vi "TriggererNot.vi"(10 "Control Name":string="Acquire Trigger", 11 "name or relative path":string="SW-Microscoper.vi") -> (0 "error out":errorcluster, 3 "VI out":refnum<vi>)   [LabVIEW 2012]
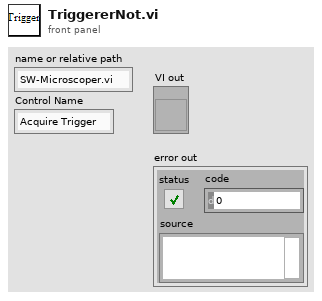
[diagram p1: front panel]
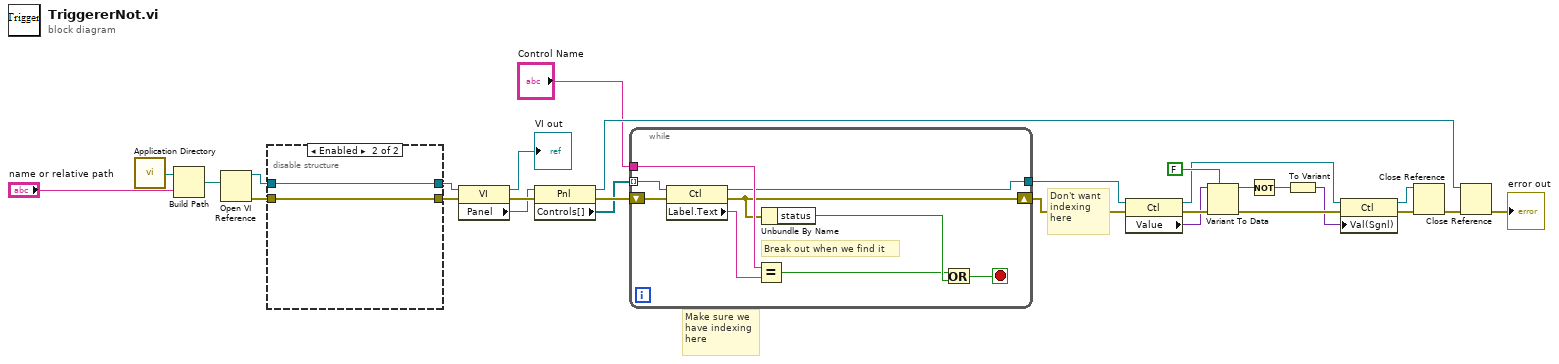
[diagram p0: block diagram]
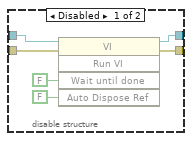
[diagram p2: hidden frame]
diagram:
  # "Don't want\nindexing\nhere"
  # "Make sure we\nhave indexing\nhere"
  n1 = call <vilib>:"Application Directory.vi"() -> ("Application Directory"=w7:path)
  n2 = Build Path(base path=w7, name or relative path="name or relative path") -> (appended path=w6:path)
  n3 = Open VI Reference(vi path=w6) -> (vi reference=w5:refnum<vi>, error out=w4:errorcluster)  [unwired: 5 in]
  n4 = disable-structure shown="Enabled" {
    disable-tunnel: w5 -> [w32 w36]
    disable-tunnel: w4 -> [w31 w35]
    disable-tunnel: [w30 w36] -> w3
    disable-tunnel: [w29 w35] -> w2
    frame Disabled {
      n5 = invoke class="VI" method="Run VI"(reference=w32, error in=w31, "Wait until done"=FALSE ("Front Panel Window:Open"), "Auto Dispose Ref"=FALSE ("Auto Dispose Reference")) -> (reference out=w30:refnum<vi>, error out=w29:errorcluster)  [unwired: 1 in, 3 out]
    }
    frame Enabled {
    }
  }
  n6 = property class="VI"(reference=w3, error in=w2) -> (reference out=→"VI out":refnum<vi>, error out=w21:errorcluster, "Panel"=w9:refnum<vi>)
  n7 = property class="Pnl"(reference=w9, error in=w21) -> (reference out=w28:refnum<vi>, error out=w22:errorcluster, "Controls[]"=w10:refnum<vi>[])
  n8 = while {
    tunnel: w10 -> [w45] mode=indexing
    tunnel: "Control Name" -> [w44]
    tunnel: [w42] -> w11
    shift-right: [w40] -> w23
    shift-left: w22 -> [w41]
    stop <- w39 stop-if-true
    # "Break out when we find it"
    n9 = property class="Ctl"(reference=w45, error in=w41) -> (reference out=w42:refnum<vi>, error out=w40:errorcluster, "Label.Text"=w43:string)
    n10 = Equal?(x=w44, y=w43) -> (x = y?=w37:bool)
    n11 = Unbundle By Name(w40) -> ("status"=w38:bool)
    n12 = Or(x=w37, y=w38) -> (x .or. y?=w39:bool)
  }
  n13 = property class="Ctl"(reference=w11, error in=w23) -> (reference out=w12:refnum<vi>, error out=w18:errorcluster, "Value"=w14:variant)
  n14 = Variant To Data(error in=w18, type=FALSE ("Push Other VI's Button 2"), Variant=w14) -> (data=w17:bool, error out=w19:errorcluster)
  n15 = Not(x=w17) -> (.not. x?=w16:bool)
  n16 = To Variant(anything=w16) -> (Variant=w13:variant)
  n17 = property class="Ctl"(reference=w12, error in=w19, "Val(Sgnl)"=w13) -> (reference out=w27:refnum<vi>, error out=w26:errorcluster)
  n18 = Close Reference(reference=w27, error in (no error)=w26) -> (error out=w24:errorcluster)
  n19 = Close Reference(reference=w28, error in (no error)=w24) -> (error out=→"error out":errorcluster)
